vi "Read States.vi"(8 "error in (no error)":errorcluster, 11 "GoToBallPlacementPositionTactic in":refnum<class "GoToBallPlacementPositionTactic.lvclass">) -> (0 "error out":errorcluster, 2 "States":T1, 3 "GoToBallPlacementPositionTactic out":refnum<class "GoToBallPlacementPositionTactic.lvclass">)   [LabVIEW 2020, in "GoToBallPlacementPositionTactic.lvclass"]
uses:
  GoToBallPlacementPositionTactic.lvclass
  StatesGoToBallPlacementPositionTactic.ctl
  GoToBallPlacementPositionTactic.lvclass/GoToBallPlacementPositionTactic.ctl
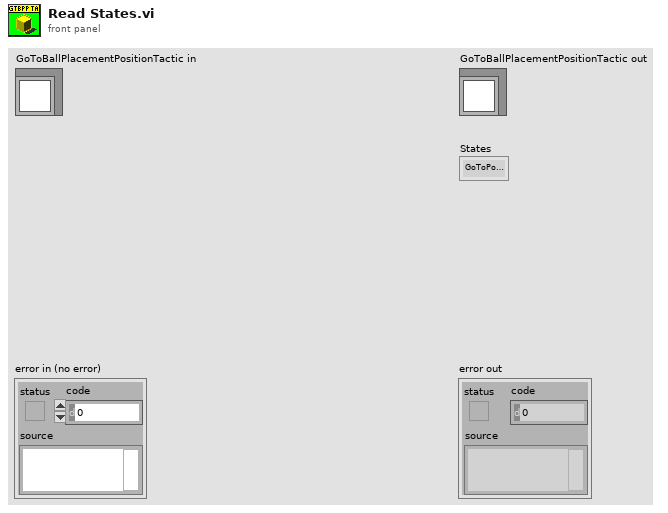
[diagram p1: front panel]
types:
  T1 = typedef "GoToBallPlacementPositionTactic.lvclass/StatesGoToBallPlacementPositionTactic.ctl" = enum16{"GoToPosition", "Exit"}
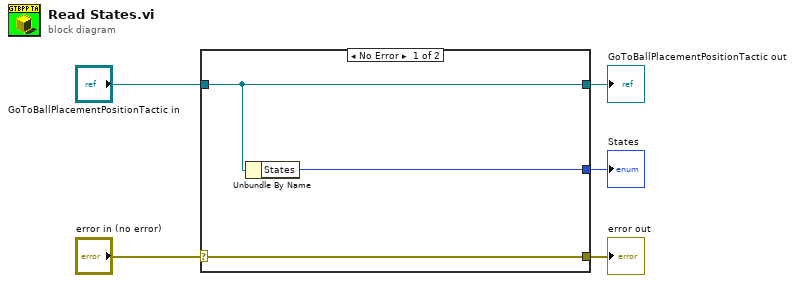
[diagram p0: block diagram]
diagram:
  n1 = case shown="No Error" "error in (no error)" {
    selector: "error in (no error)" -> [w8 w9]
    tunnel: [w8 w9] -> w4
    tunnel: [w7 w10] -> w2
    tunnel: "GoToBallPlacementPositionTactic in" -> [w7 w10]
    tunnel: [w6 _] -> w1
    frame No Error {
      n2 = Unbundle By Name(w7) -> ("States"=w6:T1)
    }
    frame Error {
    }
  }
  "error out" <- w4
  "GoToBallPlacementPositionTactic out" <- w2
  "States" <- w1
